vi "FilterInvalidCtrlRef.vi"(1 "Ctrls in":refnum<vi>[](array[refnum])) -> (0 "Ctrl out":refnum<vi>[](array[refnum]))   [LabVIEW 2018]
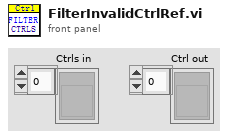
[diagram p1: front panel]
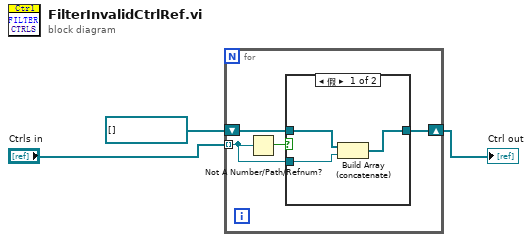
[diagram p0: block diagram]
diagram:
  n1 = for {
    tunnel: "Ctrls in" -> [w6] mode=indexing
    shift-right: [w5] -> w3
    shift-left: refnum<vi>[] [] -> [w4]
    n2 = Not A Number/Path/Refnum?(number/path/refnum=w6) -> (NaN/Path/Refnum?=w7:bool)
    n3 = case shown="假" w7 {
      tunnel: w6 -> [w10 _]
      tunnel: [w9 w11] -> w5
      tunnel: w4 -> [w8 w11]
      frame False {
        n4 = Build Array (concatenate)(w8, w10) -> (w9:refnum<vi>[])
      }
      frame True {
      }
    }
  }
  "Ctrl out" <- w3
